vi "Device Params Global.vi"(7 "action":T27, 8 "error in":errorcluster, 10 "Device Connections IN":T1={"Detector"={"Detector Type"=enum."INL PID", "Connection"=FALSE, "B-M PID"={"AI DAQmx channel"=""}, "INL PID Connections"={"PIDs"=1, "Integrator DAQ Channels 1"={"V0"="cDAQ1Mod1/ai0", "S1"="cDAQ1Mod5/port0/line4", "S2"="cDAQ1Mod5/ctr0"}, "Integrator DAQ Channels 2"={"V0"="cDAQ1Mod1/ai0", "S1"="cDAQ1Mod5/port0/line4", "S2"="cDAQ1Mod5/ctr0"}}}, "Power Supply"={"Type"=enum."Stanford Research PS350", "Connection"=FALSE, "VISA resource name"=""}, "Mass Flow Controller"={"Type"=enum."Aalborg GFC17", "Connection"=FALSE, "Aalborg GFC17"={"flow rate setpoint channel"="cDAQ1Mod3/ao0", "flow rate reading channel"="cDAQ1Mod1/ai4", "valve channel"="cDAQ1Mod3/ao1"}}, "Valve Controller"={"Type"=enum."SMC - INL", "Connection"=FALSE, "SMC - INL"={"VISA resource name"="COM3"}}, "Multimeter"={"Multimeter Type"=enum."Agilent 3458A", "Connection"=FALSE, "VISA resource name"=""}, "Vapour Generator"={"Type"=enum."Owlstone GEN-SYS", "Connection"=FALSE, "Owlstone Gen-SYS"={"GEN-SYS VISA resource name"="", "OVG-4"={"Flow Address"=2, "Temp Address"=1}, "OHG-4"={"Flow Address"=2, "Easydew VISA resource name"=""}}}} {"Detector"."INL PID Connections"."PIDs" min=1 max=2 step=1}, 11 "Device Settings IN":T11={"PID"={"B-M PID"={"Detector Sampling Frequency"=0.0}, "INL PID"={"Sampling Frequency"=0.5, "Integration Time"=50.0, "Integration Periods"=50, "Grid Voltage"=50.0}}, "Power Supply"={"Source Value"=0.0, "Source Value Units"=enum."volts", "Source Mode"=enum."Volts", "Limits"={"Voltage Limit"=0.0, "Voltage Limit Units"=enum."volts", "Current Limit"=0.0, "Current Limit Units"=enum."amps", "Voltage Trip/Cmpl"=0.0, "Voltage Trip/Cmpl Units"=enum."volts", "Current Trip/Cmpl"=0.0, "Current Trip/Cmpl Units"=enum."amps"}, "Output"=FALSE}, "Mass Flow Controller"={"MFC Flow Rate"=0.0, "MFC Valve Status"=enum."Open"}, "Valve Controller"={"Valve Assembly"={"Valve 1"=0, "Valve 2"=0, "Valve 3"=0, "Valve 4"=0, "Valve 5"=0}}, "Multimeter"={"Agilent 3458A"={"Measurement Configuration"={"Function"=enum."2-Wire Resistance", " Manual Resolution"=enum."6.5", "Frequency Source"=enum."AC Voltage", "Auto Range"=enum."ON"}, "Measurement Integration"={"Power Line Cycles"=0.0}}}, "Vapour Generator"={"Owlstone Permeation Tube"={"Tube"=enum."Isobutylene 27 Nov 2012", "Molecular Weight"=0.0, "Calibration Temperature\n(Celcius)"=0, "Permeation Rate \n(ng/min)"=0}, "Owlstone GEN-SYS Setpoints"={"OVG-4"={"Oven Temperature"=0, "Sample Flow Rate"=0, "Split Flow Status"=0, "Split Flow Rate"=0}, "OHG-4"={"Wet Air Flow"=0}}}} {"Vapour Generator"."Owlstone GEN-SYS Setpoints"."OHG-4"."Wet Air Flow" min=300 max=3000 scale=300.0..3000.0; "Vapour Generator"."Owlstone GEN-SYS Setpoints"."OVG-4"."Split Flow Status" items=["Closed", "Open"]; "Vapour Generator"."Owlstone GEN-SYS Setpoints"."OVG-4"."Split Flow Rate" min=300 max=3000 scale=50.0..3000.0; "Vapour Generator"."Owlstone GEN-SYS Setpoints"."OVG-4"."Sample Flow Rate" min=50 max=500 scale=50.0..500.0; "Vapour Generator"."Owlstone GEN-SYS Setpoints"."OVG-4"."Oven Temperature" min=25 max=100 scale=25.0..100.0; "Vapour Generator"."Owlstone Permeation Tube"."Molecular Weight" min=0.0 format="%#_3g"; "Vapour Generator"."Owlstone Permeation Tube"."Permeation Rate \n(ng/min)" min=0; "Vapour Generator"."Owlstone Permeation Tube"."Calibration Temperature\n(Celcius)" min=0; "Valve Controller"."Valve Assembly"."Valve 5" items=["Closed", "Open"]; "Valve Controller"."Valve Assembly"."Valve 4" items=["Closed", "Open"]; "Valve Controller"."Valve Assembly"."Valve 3" items=["Closed", "Open"]; "Valve Controller"."Valve Assembly"."Valve 2" items=["Closed", "Open"]; "Valve Controller"."Valve Assembly"."Valve 1" items=["Closed", "Open"]}) -> (0 "error out":errorcluster, 2 "Device Connections OUT":T1={"Detector"={"Detector Type"=enum."INL PID", "Connection"=FALSE, "B-M PID"={"AI DAQmx channel"=""}, "INL PID Connections"={"PIDs"=1, "Integrator DAQ Channels 1"={"V0"="cDAQ1Mod1/ai0", "S1"="cDAQ1Mod5/port0/line4", "S2"="cDAQ1Mod5/ctr0"}, "Integrator DAQ Channels 2"={"V0"="cDAQ1Mod1/ai0", "S1"="cDAQ1Mod5/port0/line4", "S2"="cDAQ1Mod5/ctr0"}}}, "Power Supply"={"Type"=enum."Stanford Research PS350", "Connection"=FALSE, "VISA resource name"=""}, "Mass Flow Controller"={"Type"=enum."Aalborg GFC17", "Connection"=FALSE, "Aalborg GFC17"={"flow rate setpoint channel"="cDAQ1Mod3/ao0", "flow rate reading channel"="cDAQ1Mod1/ai4", "valve channel"="cDAQ1Mod3/ao1"}}, "Valve Controller"={"Type"=enum."SMC - INL", "Connection"=FALSE, "SMC - INL"={"VISA resource name"="COM3"}}, "Multimeter"={"Multimeter Type"=enum."Agilent 3458A", "Connection"=FALSE, "VISA resource name"=""}, "Vapour Generator"={"Type"=enum."Owlstone GEN-SYS", "Connection"=FALSE, "Owlstone Gen-SYS"={"GEN-SYS VISA resource name"="", "OVG-4"={"Flow Address"=2, "Temp Address"=1}, "OHG-4"={"Flow Address"=2, "Easydew VISA resource name"=""}}}} {"Detector"."INL PID Connections"."PIDs" min=1 max=2 step=1}, 3 "Device Settings OUT":T11={"PID"={"B-M PID"={"Detector Sampling Frequency"=0.0}, "INL PID"={"Sampling Frequency"=0.5, "Integration Time"=50.0, "Integration Periods"=50, "Grid Voltage"=50.0}}, "Power Supply"={"Source Value"=0.0, "Source Value Units"=enum."volts", "Source Mode"=enum."Volts", "Limits"={"Voltage Limit"=0.0, "Voltage Limit Units"=enum."volts", "Current Limit"=0.0, "Current Limit Units"=enum."amps", "Voltage Trip/Cmpl"=0.0, "Voltage Trip/Cmpl Units"=enum."volts", "Current Trip/Cmpl"=0.0, "Current Trip/Cmpl Units"=enum."amps"}, "Output"=FALSE}, "Mass Flow Controller"={"MFC Flow Rate"=0.0, "MFC Valve Status"=enum."Open"}, "Valve Controller"={"Valve Assembly"={"Valve 1"=0, "Valve 2"=0, "Valve 3"=0, "Valve 4"=0, "Valve 5"=0}}, "Multimeter"={"Agilent 3458A"={"Measurement Configuration"={"Function"=enum."2-Wire Resistance", " Manual Resolution"=enum."6.5", "Frequency Source"=enum."AC Voltage", "Auto Range"=enum."ON"}, "Measurement Integration"={"Power Line Cycles"=0.0}}}, "Vapour Generator"={"Owlstone Permeation Tube"={"Tube"=enum."Isobutylene 27 Nov 2012", "Molecular Weight"=0.0, "Calibration Temperature\n(Celcius)"=0, "Permeation Rate \n(ng/min)"=0}, "Owlstone GEN-SYS Setpoints"={"OVG-4"={"Oven Temperature"=0, "Sample Flow Rate"=0, "Split Flow Status"=0, "Split Flow Rate"=0}, "OHG-4"={"Wet Air Flow"=0}}}} {"Vapour Generator"."Owlstone GEN-SYS Setpoints"."OHG-4"."Wet Air Flow" min=300 max=3000 scale=300.0..3000.0; "Vapour Generator"."Owlstone GEN-SYS Setpoints"."OVG-4"."Split Flow Status" items=["Closed", "Open"]; "Vapour Generator"."Owlstone GEN-SYS Setpoints"."OVG-4"."Split Flow Rate" min=300 max=3000 scale=50.0..3000.0; "Vapour Generator"."Owlstone GEN-SYS Setpoints"."OVG-4"."Sample Flow Rate" min=50 max=500 scale=50.0..500.0; "Vapour Generator"."Owlstone GEN-SYS Setpoints"."OVG-4"."Oven Temperature" min=25 max=100 scale=25.0..100.0; "Vapour Generator"."Owlstone Permeation Tube"."Molecular Weight" min=0.0 format="%#_3g"; "Vapour Generator"."Owlstone Permeation Tube"."Permeation Rate \n(ng/min)" min=0; "Vapour Generator"."Owlstone Permeation Tube"."Calibration Temperature\n(Celcius)" min=0; "Valve Controller"."Valve Assembly"."Valve 5" items=["Closed", "Open"]; "Valve Controller"."Valve Assembly"."Valve 4" items=["Closed", "Open"]; "Valve Controller"."Valve Assembly"."Valve 3" items=["Closed", "Open"]; "Valve Controller"."Valve Assembly"."Valve 2" items=["Closed", "Open"]; "Valve Controller"."Valve Assembly"."Valve 1" items=["Closed", "Open"]})   [LabVIEW 2011]
uses:
  Device Params Global.ctl
  Controls/Device Settings.ctl
  Modules/Hardware/Baseline Mocon piD-Tech plus/Settings.ctl
  Modules/Hardware/INL PID/Settings.ctl
  Modules/Hardware/Power Supply/Source Units.ctl
  Modules/Hardware/Power Supply/Source Mode.ctl
  Modules/Hardware/Power Supply/Protection Limits.ctl
  Modules/Hardware/Power Supply/Voltage Units.ctl
  Modules/Hardware/Power Supply/Current Units.ctl
  Modules/Hardware/Mass Flow Controller/Valve Status.ctl
  Modules/Hardware/Valve Controller/Valve Assembly.ctl
  Modules/Hardware/Valve Controller/Status.ctl
  Modules/Hardware/Agilent 3458A/Measurement Configuration.ctl
  Modules/Hardware/Agilent 3458A/Measurement Integration.ctl
  Modules/Hardware/Owlstone GEN-SYS/Permeation Tube.ctl
  Modules/Hardware/Owlstone GEN-SYS/Permeation Tube Gas.ctl
  Modules/Hardware/Owlstone GEN-SYS/Gen-Sys Setpoints.ctl
  Controls/Device Connections.ctl
  Controls/Detector Type.ctl
  Modules/Hardware/Baseline Mocon piD-Tech plus/Connections.ctl
  Controls/INL PID Connections.ctl
  Modules/Hardware/INL PID/Integrator DAQmx Channels.ctl
  Modules/Hardware/Aalborg GFC17/Aalborg GFC17 Connections.ctl
  Controls/Valve Type.ctl
  Controls/Multimeter Type.ctl
  Controls/Vapour Generator Type.ctl
  Modules/Hardware/Owlstone GEN-SYS/GEN-SYS Connections.ctl
  Modules/Hardware/Mass Flow Controller/Mass Flow Controller.lvclass
  Modules/Hardware/Power Supply/Power Supply.lvclass
  Modules/Hardware/INL PID/INL PID.lvclass
  Modules/Hardware/Valve Controller/Valve Controller.lvclass
  Modules/Hardware/Aalborg GFC17/Aalborg GFC17.lvclass
  Modules/Hardware/Agilent 3458A/Agilent 3458A.lvclass
  Modules/Hardware/Owlstone GEN-SYS/Owlstone GEN-SYS.lvclass
  Modules/Hardware/Baseline Mocon piD-Tech plus/Baseline Mocon piD-Tech plus.lvclass
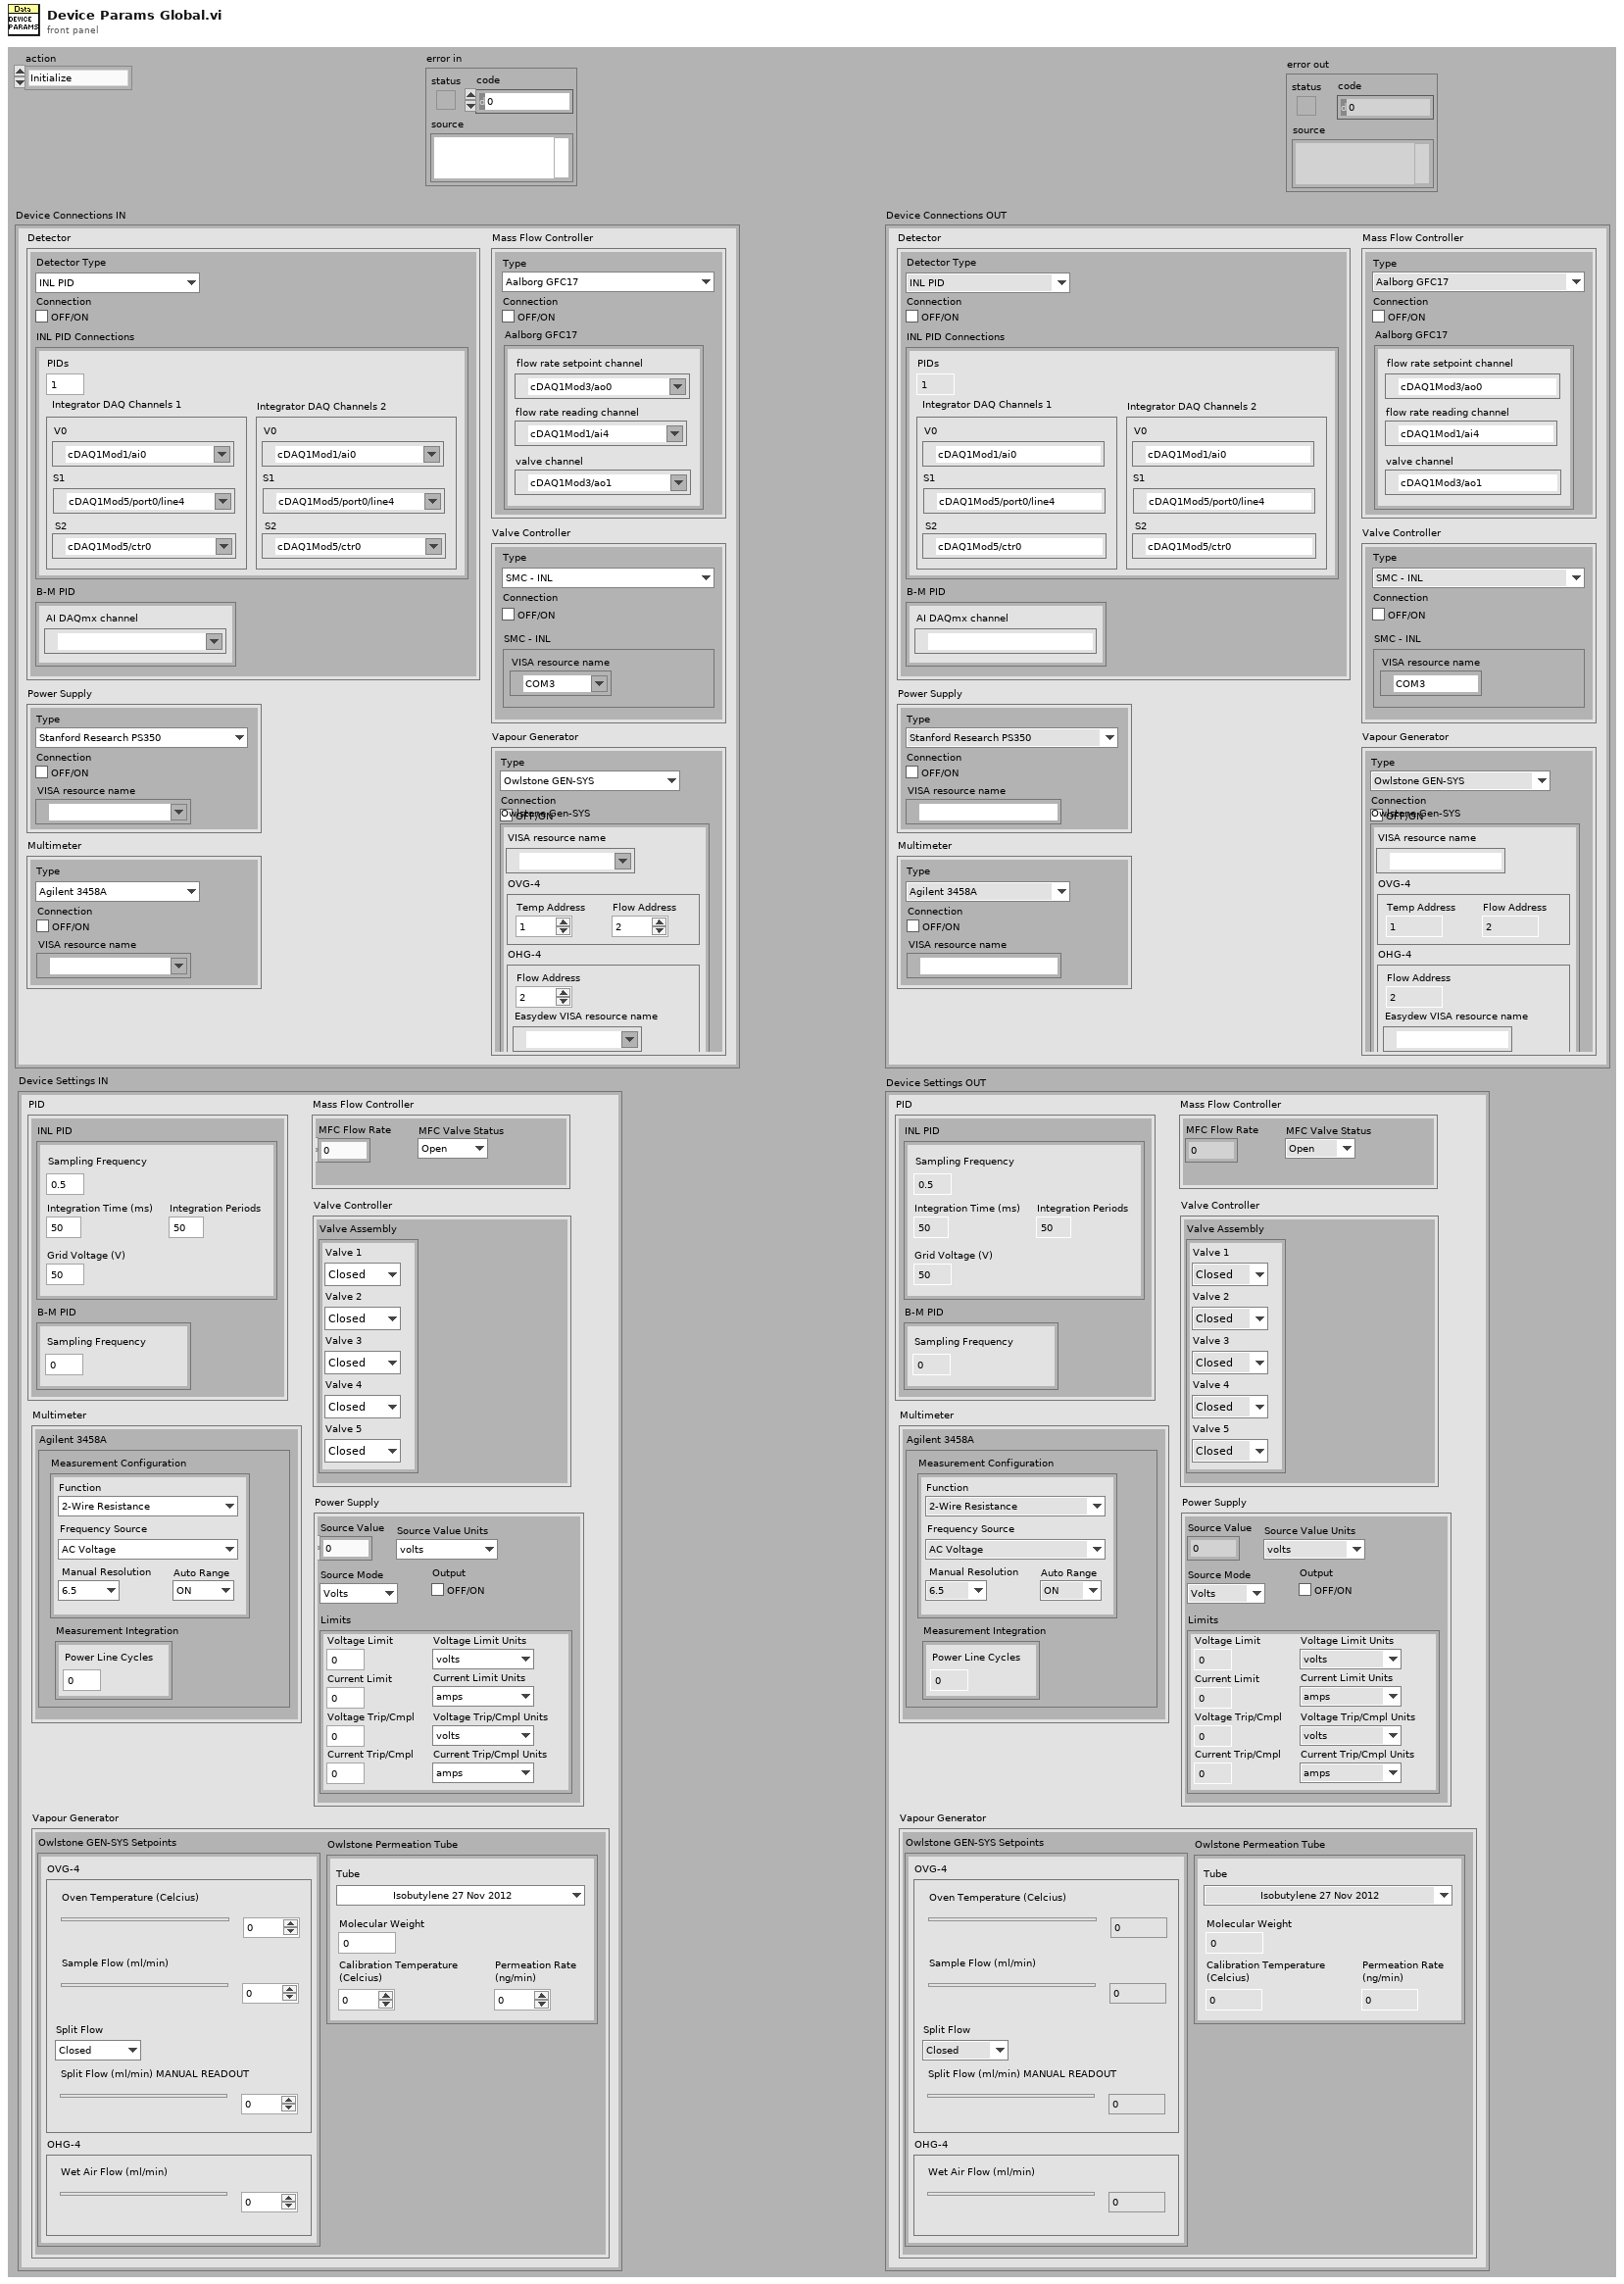
[diagram p1: front panel]
types:
  T1 = typedef "Device Connections.ctl" = cluster{"Detector":cluster{"Detector Type":T2, "Connection":bool, "B-M PID":T3, "INL PID Connections":T4}, "Power Supply":cluster{"Type":enum16{"Stanford Research PS350", "Keithley 2400"}, "Connection":bool, "VISA resource name":refnum<visa-resource-name>}, "Mass Flow Controller":cluster{"Type":enum16{"Aalborg GFC17"}, "Connection":bool, "Aalborg GFC17":T6}, "Valve Controller":cluster{"Type":T7, "Connection":bool, "SMC - INL":cluster{"VISA resource name":refnum<visa-resource-name>}}, "Multimeter":cluster{"Multimeter Type":T8, "Connection":bool, "VISA resource name":refnum<visa-resource-name>}, "Vapour Generator":cluster{"Type":T9, "Connection":bool, "Owlstone Gen-SYS":T10}}
  T2 = typedef "Detector Type.ctl" = enum16{"INL PID", "Baseline-Mocon piD-TECH plus"}
  T3 = typedef "Baseline Mocon piD-Tech plus.lvclass/Connections.ctl" = cluster{"AI DAQmx channel":tag}
  T4 = typedef "INL PID Connections.ctl" = cluster{"PIDs":u8, "Integrator DAQ Channels 1":T5, "Integrator DAQ Channels 2":T5}
  T5 = typedef "INL PID.lvclass/Integrator DAQmx Channels.ctl" = cluster{"V0":tag, "S1":tag, "S2":tag}
  T6 = typedef "Aalborg GFC17.lvclass/Aalborg GFC17 Connections.ctl" = cluster{"flow rate setpoint channel":tag, "flow rate reading channel":tag, "valve channel":tag}
  T7 = typedef "Valve Type.ctl" = enum16{"SMC - INL"}
  T8 = typedef "Multimeter Type.ctl" = enum16{"Agilent 3458A"}
  T9 = typedef "Vapour Generator Type.ctl" = enum16{"Owlstone GEN-SYS"}
  T10 = typedef "Owlstone GEN-SYS.lvclass/GEN-SYS Connections.ctl" = cluster{"GEN-SYS VISA resource name":refnum<visa-resource-name>, "OVG-4":cluster{"Flow Address":u8, "Temp Address":u8}, "OHG-4":cluster{"Flow Address":u8, "Easydew VISA resource name":refnum<visa-resource-name>}}
  T11 = typedef "Device Settings.ctl" = cluster{"PID":cluster{"B-M PID":T12, "INL PID":T13}, "Power Supply":cluster{"Source Value":dbl, "Source Value Units":T14, "Source Mode":T15, "Limits":T16, "Output":bool}, "Mass Flow Controller":cluster{"MFC Flow Rate":dbl, "MFC Valve Status":T19}, "Valve Controller":cluster{"Valve Assembly":T20}, "Multimeter":cluster{"Agilent 3458A":cluster{"Measurement Configuration":T22, "Measurement Integration":T23}}, "Vapour Generator":cluster{"Owlstone Permeation Tube":T24, "Owlstone GEN-SYS Setpoints":T26}}
  T12 = typedef "Baseline Mocon piD-Tech plus.lvclass/Settings.ctl" = cluster{"Detector Sampling Frequency":dbl}
  T13 = typedef "INL PID.lvclass/Settings.ctl" = cluster{"Sampling Frequency":dbl, "Integration Time":dbl, "Integration Periods":u8, "Grid Voltage":dbl}
  T14 = typedef "Power Supply.lvclass/Source Units.ctl" = enum16{"volts", "millivolts", "microvolts", "amps", "milliamps", "microamps", "nanoamps"}
  T15 = typedef "Power Supply.lvclass/Source Mode.ctl" = enum16{"Volts", "Current"}
  T16 = typedef "Power Supply.lvclass/Protection Limits.ctl" = cluster{"Voltage Limit":dbl, "Voltage Limit Units":T17, "Current Limit":dbl, "Current Limit Units":T18, "Voltage Trip/Cmpl":dbl, "Voltage Trip/Cmpl Units":T17, "Current Trip/Cmpl":dbl, "Current Trip/Cmpl Units":T18}
  T17 = typedef "Power Supply.lvclass/Voltage Units.ctl" = enum16{"volts", "millivolts", "microvolts"}
  T18 = typedef "Power Supply.lvclass/Current Units.ctl" = enum16{"amps", "milliamps", "microamps", "nanoamps"}
  T19 = typedef "Mass Flow Controller.lvclass/Valve Status.ctl" = enum16{"Open", "Closed"}
  T20 = typedef "Valve Controller.lvclass/Valve Assembly.ctl" = cluster{"Valve 1":T21, "Valve 2":T21, "Valve 3":T21, "Valve 4":T21, "Valve 5":T21}
  T21 = typedef "Valve Controller.lvclass/Status.ctl" = u16
  T22 = typedef "Agilent 3458A.lvclass/Measurement Configuration.ctl" = cluster{"Function":enum16{"DC Voltage", "AC Voltage", "AC + DC Voltage", "DC Current", "AC Current", "AC + DC Current", "2-Wire Resistance", "4-Wire Resistance", "Frequency", "Period", "Direct Sampling DC", "Direct Sampling AC", "Sub-Sampling DC", "Sub-Sampling AC"}, " Manual Resolution":enum16{"4.5", "5.5", "6.5", "7.5", "8.5"}, "Frequency Source":enum16{"AC + DC Current", "AC + DC Voltage", "AC Current", "AC Voltage"}, "Auto Range":enum16{"OFF", "ON", "ONCE"}}
  T23 = typedef "Agilent 3458A.lvclass/Measurement Integration.ctl" = cluster{"Power Line Cycles":dbl}
  T24 = typedef "Owlstone GEN-SYS.lvclass/Permeation Tube.ctl" = cluster{"Tube":T25, "Molecular Weight":dbl, "Calibration Temperature\n(Celcius)":i32, "Permeation Rate \n(ng/min)":i32}
  T25 = typedef "Owlstone GEN-SYS.lvclass/Permeation Tube Gas.ctl" = enum16{"Isobutylene 27 Nov 2012", "Ammonia 29 Sep 2012", "DMMP Tube A 3 July 2014", "DMMP Tube B 3 July 2014"}
  T26 = typedef "Owlstone GEN-SYS.lvclass/Gen-Sys Setpoints.ctl" = cluster{"OVG-4":cluster{"Oven Temperature":i32, "Sample Flow Rate":i32, "Split Flow Status":u16, "Split Flow Rate":i32}, "OHG-4":cluster{"Wet Air Flow":i32}}
  T27 = typedef "Device Params Global.ctl" = enum16{"Initialize", "Get Device Settings", "Get Device Connections", "Set Device Settings", "Set Device Connections", "Get All Device Properties"}
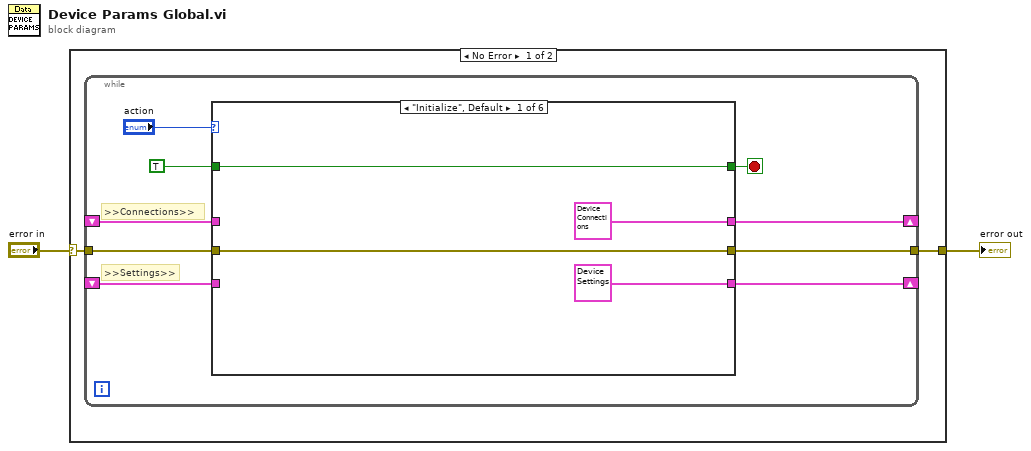
[diagram p0: block diagram]
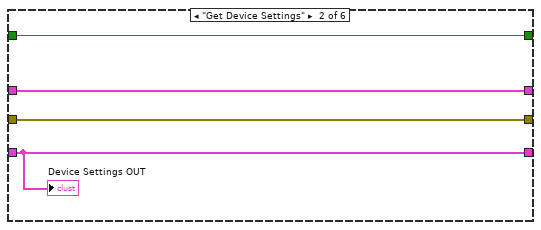
[diagram p2: hidden frame]
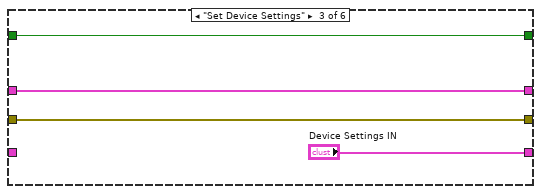
[diagram p3: hidden frame]
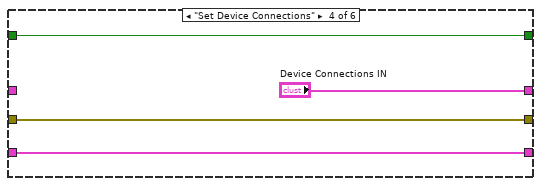
[diagram p4: hidden frame]
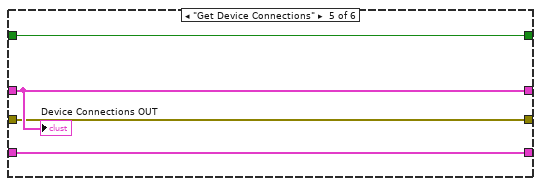
[diagram p5: hidden frame]
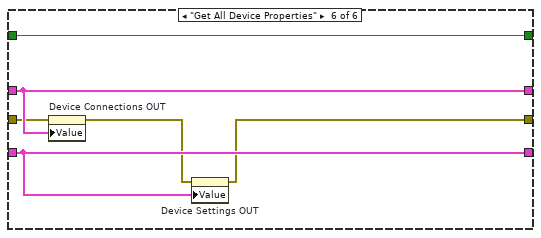
[diagram p6: hidden frame]
diagram:
  n1 = case shown="No Error" "error in" {
    selector: "error in" -> [w4 w40]
    tunnel: [w3 w40] -> w1
    frame No Error {
      n2 = while {
        tunnel: w4 -> [w12]
        tunnel: [w11] -> w3
        shift-right: [w9] -> _
        shift-left: _ -> [w8]
        shift-right: [w6] -> _
        shift-left: _ -> [w7]
        stop <- w10 stop-if-true
        # ">>Settings>>"
        # ">>Connections>>"
        n3 = case shown="\"Initialize\", Default" "action" {
          tunnel: w12 -> [w17 w21 w25 w27 w31 w38]
          tunnel: [w17 w21 w25 w27 w31 w35] -> w11
          tunnel: [w14 w18 w22 w26 w30 w34] -> w10
          tunnel: [T11 {"PID"={"B-M PID"={"Detector Sampling Frequency"=0.0}, "INL PID"={"Sampling Frequency"=0.0, "Integration Time"=0.0, "Integration Periods"=0, "Grid Voltage"=0.0}}, "Power Supply"={"Source Value"=0.0, "Source Value Units"=enum."volts", "Source Mode"=enum."Volts", "Limits"={"Voltage Limit"=0.0, "Voltage Limit Units"=enum."volts", "Current Limit"=0.0, "Current Limit Units"=enum."amps", "Voltage Trip/Cmpl"=0.0, "Voltage Trip/Cmpl Units"=enum."volts", "Current Trip/Cmpl"=0.0, "Current Trip/Cmpl Units"=enum."amps"}, "Output"=FALSE}, "Mass Flow Controller"={"MFC Flow Rate"=0.0, "MFC Valve Status"=enum."Open"}, "Valve Controller"={"Valve Assembly"={"Valve 1"=0, "Valve 2"=0, "Valve 3"=0, "Valve 4"=0, "Valve 5"=0}}, "Multimeter"={"Agilent 3458A"={"Measurement Configuration"={"Function"=enum."DC Voltage", " Manual Resolution"=enum."4.5", "Frequency Source"=enum."AC + DC Current", "Auto Range"=enum."OFF"}, "Measurement Integration"={"Power Line Cycles"=0.0}}}, "Vapour Generator"={"Owlstone Permeation Tube"={"Tube"=enum."Isobutylene 27 Nov 2012", "Molecular Weight"=0.0, "Calibration Temperature\n(Celcius)"=0, "Permeation Rate \n(ng/min)"=0}, "Owlstone GEN-SYS Setpoints"={"OVG-4"={"Oven Temperature"=0, "Sample Flow Rate"=0, "Split Flow Status"=0, "Split Flow Rate"=0}, "OHG-4"={"Wet Air Flow"=0}}}} ("Device Settings") w20 "Device Settings IN" w28 w32 w37] -> w9
          tunnel: w8 -> [_ w20 _ w28 w32 w37]
          tunnel: [T1 {"Detector"={"Detector Type"=enum."INL PID", "Connection"=FALSE, "B-M PID"={"AI DAQmx channel"=""}, "INL PID Connections"={"PIDs"=0, "Integrator DAQ Channels 1"={"V0"="", "S1"="", "S2"=""}, "Integrator DAQ Channels 2"={"V0"="", "S1"="", "S2"=""}}}, "Power Supply"={"Type"=enum."Stanford Research PS350", "Connection"=FALSE, "VISA resource name"=""}, "Mass Flow Controller"={"Type"=enum."Aalborg GFC17", "Connection"=FALSE, "Aalborg GFC17"={"flow rate setpoint channel"="", "flow rate reading channel"="", "valve channel"=""}}, "Valve Controller"={"Type"=enum."SMC - INL", "Connection"=FALSE, "SMC - INL"={"VISA resource name"=""}}, "Multimeter"={"Multimeter Type"=enum."Agilent 3458A", "Connection"=FALSE, "VISA resource name"=""}, "Vapour Generator"={"Type"=enum."Owlstone GEN-SYS", "Connection"=FALSE, "Owlstone Gen-SYS"={"GEN-SYS VISA resource name"="", "OVG-4"={"Flow Address"=0, "Temp Address"=0}, "OHG-4"={"Flow Address"=0, "Easydew VISA resource name"=""}}}} ("Device Connections IN") w19 w23 "Device Connections IN" w33 w39] -> w6
          tunnel: w7 -> [_ w19 w23 _ w33 w39]
          tunnel: TRUE -> [w14 w18 w22 w26 w30 w34]
          frame "Initialize", Default {
          }
          frame "Get Device Settings" {
            "Device Settings OUT" <- w20
          }
          frame "Set Device Settings" {
          }
          frame "Set Device Connections" {
          }
          frame "Get Device Connections" {
            "Device Connections OUT" <- w33
          }
          frame "Get All Device Properties" {
            n4 = property on="Device Connections OUT" class="Clust (strict)"(error in=w38, "Value"=w39) -> (error out=w36:errorcluster)  [unwired: 1 in, 1 out]
            n5 = property on="Device Settings OUT" class="Clust (strict)"(error in=w36, "Value"=w37) -> (error out=w35:errorcluster)  [unwired: 1 in, 1 out]
          }
        }
      }
    }
    frame Error {
    }
  }
  "error out" <- w1
